vi "UpdateData.vi"(8 "error in (no error)":errorcluster, 10 "Select Conditions Criteria":T1, 11 "object in":refnum<class "TableLogger_SQLite_Actor.lvclass">) -> (0 "error out":errorcluster, 2 "Data Clusters":variant[](array[variant]), 3 "object out":refnum<class "TableLogger_SQLite_Actor.lvclass">)   [LabVIEW 2014, in "TableLogger_SQLite_Actor.lvlib" / "TableLogger_SQLite_Actor.lvclass"]
uses:
  TableLogger_SQLite_Actor.lvclass
  TableLogger_Actor/SelectConditionCriteria.ctl
  SelectConditions.ctl
  TableLogger_SQLite_Actor.lvclass/TableLogger_SQLite_Actor.ctl
  <vilib>/drjdpowell/SQLite Library/SQL Connection/Execute SQL.vi
  <vilib>/drjdpowell/SQLite Library/SQLite.lvlib
  TableLogger_Actor/TableLogger_Actor/TableLogger_Actor.lvclass
  <vilib>/drjdpowell/SQLite Library/SQL Connection/Connection.lvclass
  TableLogger_Actor/TableLogger_Actor.lvlib
panel:
  # "Connector Pane"
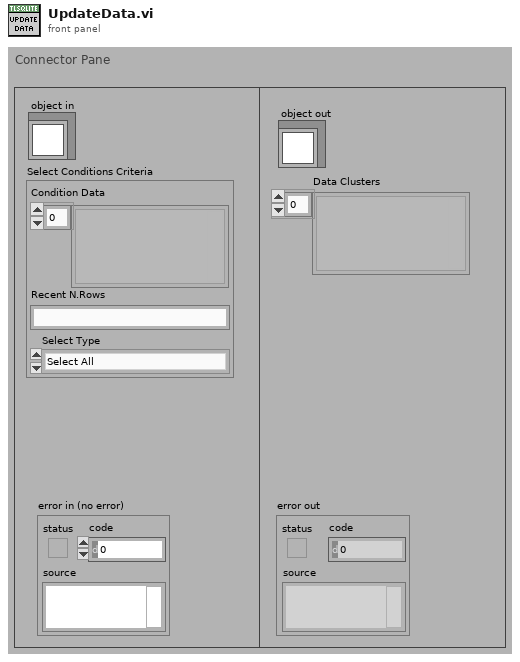
[diagram p1: front panel]
types:
  T1 = typedef "TableLogger_Actor.lvlib/SelectConditionCriteria.ctl" = cluster{"Condition Data":variant[], "Recent N.Rows":string, "Select Type":T2}
  T2 = typedef "TableLogger_Actor.lvlib/SelectConditions.ctl" = enum16{"Select All", "Select with AND Operator", "Select Most Recent Rows", "Select with OR Operator", "Select with BETWEEN Operator"}
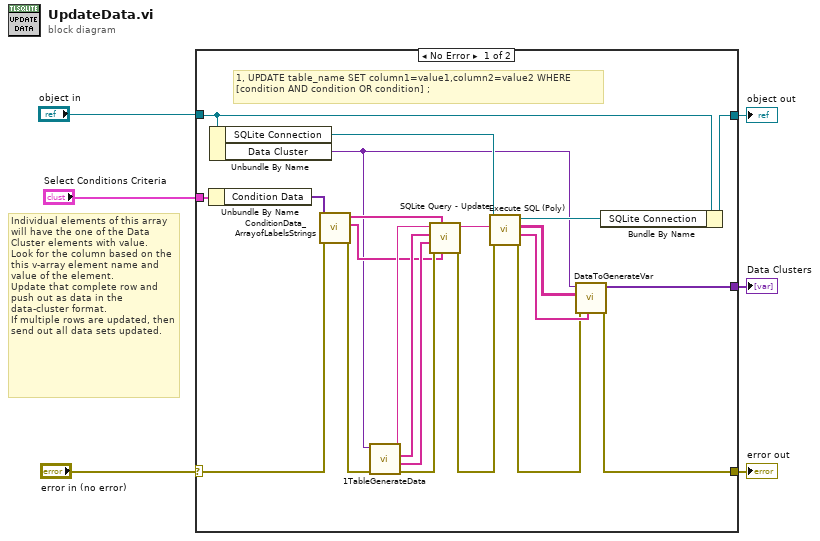
[diagram p0: block diagram]
diagram:
  # "Individual elements of this array will have the one of the Data Cluster elements with value.\nLook for the column based on the this v-array element name and value of the element.\nUpdate that complete row and push out as data in the data-cluster format.\nIf multiple rows are updated, then send out all data sets updated."
  n1 = case shown="No Error" "error in (no error)" {
    selector: "error in (no error)" -> [w18 w30]
    tunnel: [w13 w30] -> w5
    tunnel: [w28 w29] -> w3
    tunnel: "object in" -> [w27 w29]
    tunnel: [w12 _] -> w2
    tunnel: "Select Conditions Criteria" -> [w9 _]
    frame No Error {
      # "1, UPDATE table_name SET column1=value1,column2=value2 WHERE [condition AND condition OR condition] ;"
      n2 = Unbundle By Name(w9) -> ("Condition Data"=w8:variant[])
      n3 = Unbundle By Name(w27) -> ("SQLite Connection"=w26:refnum<class "Connection.lvclass">, "Data Cluster"=w7:variant)
      n4 = call "ConditionData_ArrayofLabelsStrings.vi"("error in (no error)"=w18, "Condition Data"=w8) -> ("error out"=w17:errorcluster, "Value"=w10:string[], "Label"=w11:string[])  [unwired: 7 in]
      n5 = call "1TableGenerateData.vi"("error in (no error)"=w17, "Cluster Variant"=w7) -> ("error out"=w22:errorcluster, "Data"=w24:string[], "Headers"=w20:string[], "Table Name"=w19:string)  [unwired: 5 in, 1 out]
      n6 = call "SQLite Query - Update.vi"("A[Strings] Value"=w10, "A[Strings]"=w11, "error in"=w22, "Data"=w24, "Table Headers"=w20, "Table Name"=w19) -> ("error out"=w21:errorcluster, "SQLite Query"=w23:string)  [unwired: 4 in]
      n7 = call-poly <vilib>:"Execute SQL (Poly).vi"("error in (no error)"=w21, "SQL"=w23, "SQLite Connection in"=w26) -> ("error out"=w14:errorcluster, "Column Names"=w15:string[], "Result Set"=w16:string[][], "SQLite Connection"=w25:refnum<class "Connection.lvclass">)  [unwired: 5 in]
      n8 = call "DataToGenerateVar.vi"("Header"=w15, "error in (no error)"=w14, "Data in"=w16, "Variant"=w7) -> ("error out"=w13:errorcluster, "Data"=w12:variant[])  [unwired: 6 in]
      n9 = Bundle By Name(cluster=w27, "SQLite Connection"=w25) -> (w28:refnum<class "TableLogger_SQLite_Actor.lvclass">)
    }
    frame Error {
    }
  }
  "error out" <- w5
  "object out" <- w3
  "Data Clusters" <- w2
